vi "Get_Beam_names.vi"(0 "String Value":string, 1 "Beam Names":string[](array[string])) -> (2 "Fixed Axis":T1, 3 "Beam Array":T2[](array[typedef]) items=["Green Unshifted", "Green Shifted", "Blue Unshifted", "Blue Shifted"], 4 "Error Comments":string)   [LabVIEW 2018]
uses:
  Controls/Beam_Type.ctl
  Gen Trav/Route mapping/Axis.ctl
panel:
  in  "Beam Type":T2 items=["Green Unshifted", "Green Shifted", "Blue Unshifted", "Blue Shifted"]
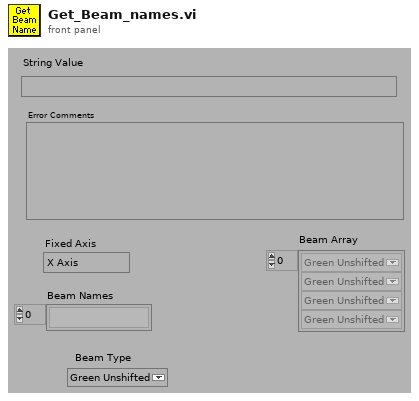
[diagram p1: front panel]
types:
  T1 = typedef "Axis.ctl" = enum16{"X Axis", "X Axis -ve", "Y Axis", "Y Axis -ve", "Z Axis", "Z Axis -ve"}
  T2 = typedef "Beam_Type.ctl" = u16
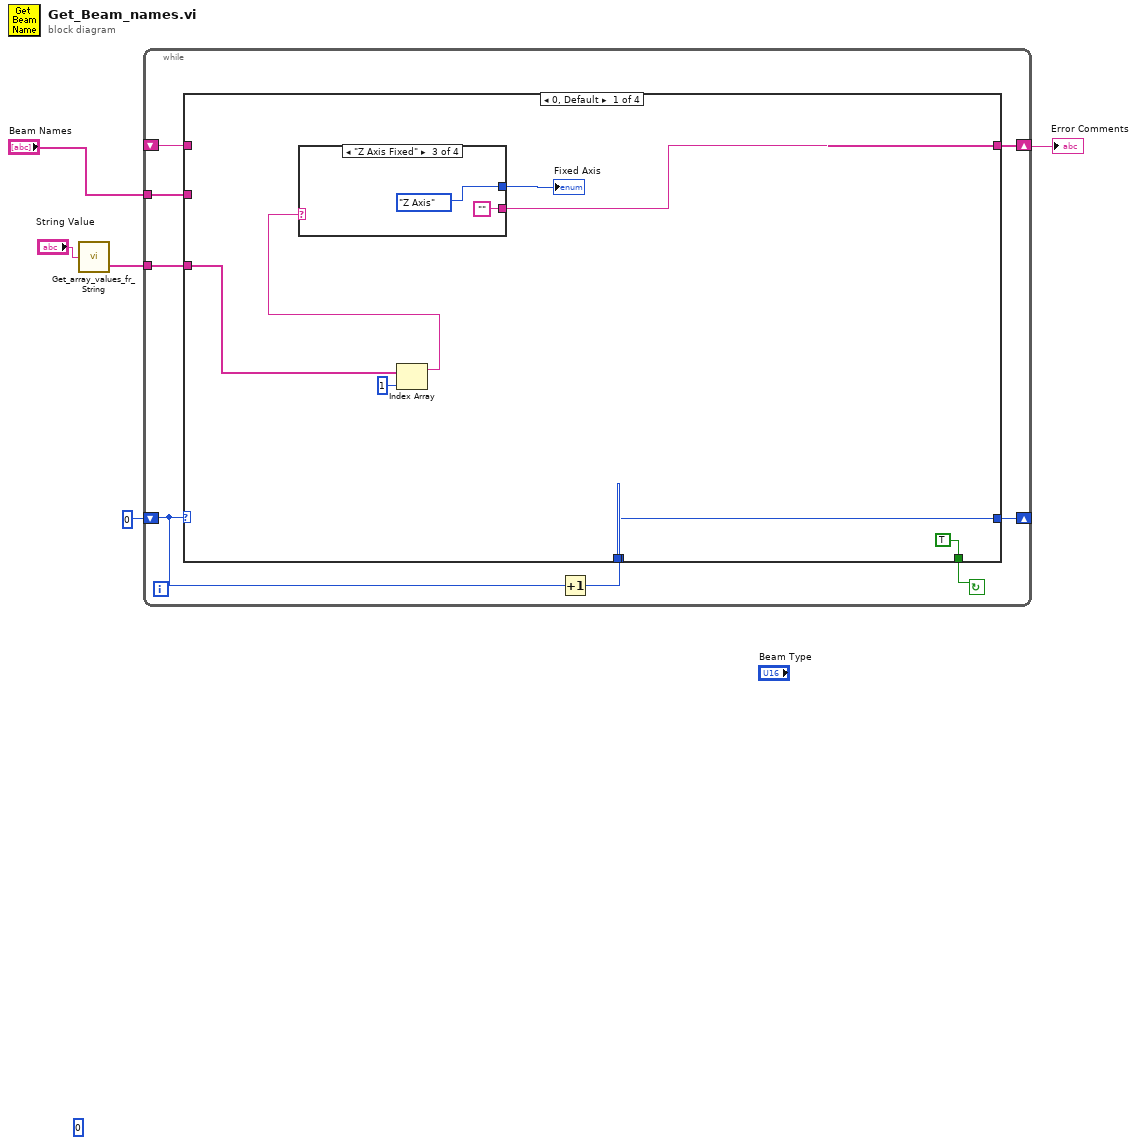
[diagram p0: block diagram]
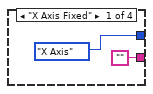
[diagram p2: hidden frame]
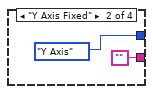
[diagram p3: hidden frame]
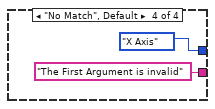
[diagram p4: hidden frame]
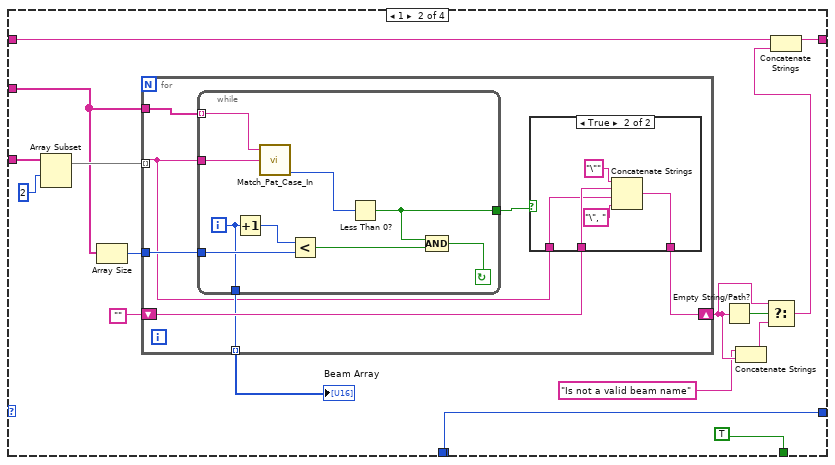
[diagram p5: hidden frame]
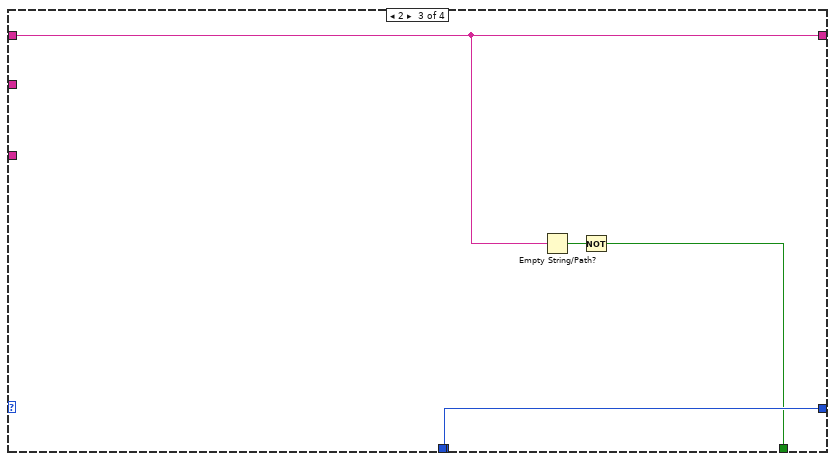
[diagram p7: hidden frame]
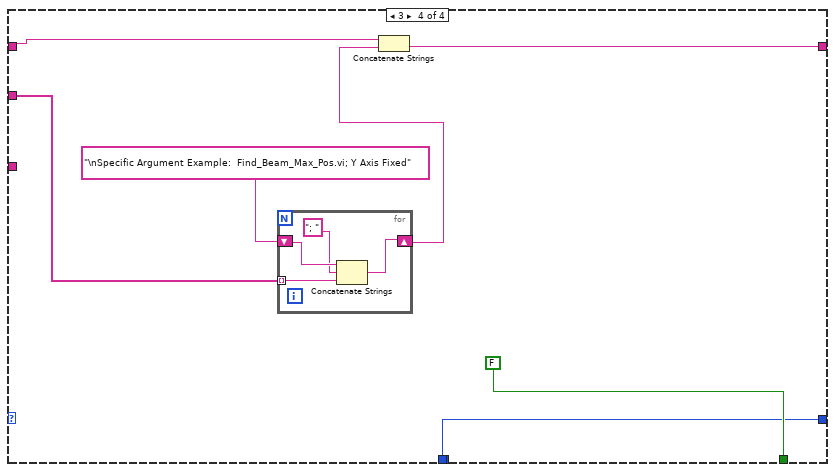
[diagram p8: hidden frame]
diagram:
  (unwired) 0 ("Index")
  n1 = call "Get_array_values_fr_String.vi"("String Value"="String Value") -> ("String array"=w2:string[])  [unwired: 1 out]
  n2 = while {
    tunnel: "Beam Names" -> [w6]
    shift-left: _ -> [w8]
    shift-right: [w9] -> w3
    tunnel: w2 -> [w13]
    shift-left: 0 -> [w12]
    shift-right: [w11] -> _
    stop <- w10 continue-if-true
    n3 = Increment(x=w12) -> (x+1=w7:i32)
    n4 = case shown="0, Default" w12 {
      tunnel: w13 -> [w19 w36 _ _]
      tunnel: w7 -> [w18 w44 w70 _]
      tunnel: [w18 w44 w70 w74] -> w11
      tunnel: [TRUE TRUE w67 FALSE] -> w10
      tunnel: [w14 w41 w69 w76] -> w9
      tunnel: w8 -> [_ w42 w69 w77]
      tunnel: w7 -> [_ _ _ w74]
      tunnel: w6 -> [_ w34 _ w72]
      frame 0, Default {
        n5 = Index Array(array=w19, index=1 ("Index")) -> (element=w15:string)
        n6 = case shown="\"Z Axis Fixed\"" w15 {
          tunnel: ["" "" "" "The First Argument is invalid"] -> w14
          tunnel: [Axis."X Axis" ("Enum") Axis."Y Axis" ("Enum") Axis."Z Axis" ("Enum") Axis."X Axis" ("Enum")] -> w16
          frame "X Axis Fixed" {
          }
          frame "Y Axis Fixed" {
          }
          frame "Z Axis Fixed" {
          }
          frame "No Match", Default {
          }
        }
        "Fixed Axis" <- w16
      }
      frame 1 {
        n7 = Array Subset(array=w36, index=2 ("Array Index")) -> (w35:string[])  [unwired: 1 in]
        n8 = Array Size(array=w34) -> (size(s)=w38:i32)
        n9 = for {
          tunnel: w34 -> [w51]
          tunnel: w35 -> [w45] mode=indexing
          tunnel: w38 -> [w50]
          shift-right: [w48] -> w31
          shift-left: "" -> [w49]
          tunnel: [w46] -> w40 mode=indexing
          n10 = while {
            tunnel: [w53] -> w46
            tunnel: [w54] -> w47
            tunnel: w50 -> [w58]
            tunnel: w45 -> [w60]
            tunnel: w51 -> [w52] mode=indexing
            i -> [w53]
            stop <- w56 continue-if-true
            n11 = Increment(x=w53) -> (x+1=w59:i32)
            n12 = call "Match_Pat_Case_In.vi"("String to match"=w52, "String"=w60) -> ("offset past match"=w55:i32)  [unwired: 1 in, 3 out]
            n13 = Less?(x=w59, y=w58) -> (x < y?=w57:bool)
            n14 = Less Than 0?(x=w55) -> (x < 0?=w54:bool)
            n15 = Compound Arithmetic op=AND(w54, w57) -> (w56:bool)
          }
          n16 = case shown="True" w47 {
            tunnel: w45 -> [_ w65]
            tunnel: w49 -> [w61 w66]
            tunnel: [w61 w64] -> w48
            frame False {
            }
            frame True {
              n17 = Concatenate Strings("\"" ("Substring"), w66, w65, "\", " ("Substring")) -> (w64:string)
            }
          }
        }
        "Beam Array" <- w40
        n18 = Empty String/Path?(string/path=w31) -> (empty?=w33:bool)
        n19 = Concatenate Strings("Is not a valid beam name" ("Substring"), w31) -> (w30:string)
        n20 = Select(t=w31, s=w33, f=w30) -> (s? t:f=w32:string)
        n21 = Concatenate Strings(w42, w32) -> (w41:string)
      }
      frame 2 {
        n22 = Empty String/Path?(string/path=w69) -> (empty?=w68:bool)
        n23 = Not(x=w68) -> (.not. x?=w67:bool)
      }
      frame 3 {
        n24 = for {
          shift-right: [w81] -> w73
          shift-left: "\nSpecific Argument Example:  Find_Beam_Max_Pos.vi; Y Axis Fixed" -> [w80]
          tunnel: w72 -> [w78] mode=indexing
          n25 = Concatenate Strings(w80, "; " ("Substring"), w78) -> (w81:string)
        }
        n26 = Concatenate Strings(w77, w73) -> (w76:string)
      }
    }
  }
  "Error Comments" <- w3
